vi "SW_BoolArryToNumber2.vi"(8 "error in (no error)":errorcluster caption="错误输入（无错误）", 10 "L32 INUPT":string="1.0.0.0", 11 "H32 INUPT":string="2.0.0.0") -> (0 "error out":errorcluster caption="错误输出", 1 "64 SW OUT":bool[](array[boolean]), 2 "L_32":bool[](array[boolean]), 3 "H_32":bool[](array[boolean]))   [LabVIEW 2018]
panel:
  out "数组 2":string[](array[string])
  out "数组":string[](array[string])
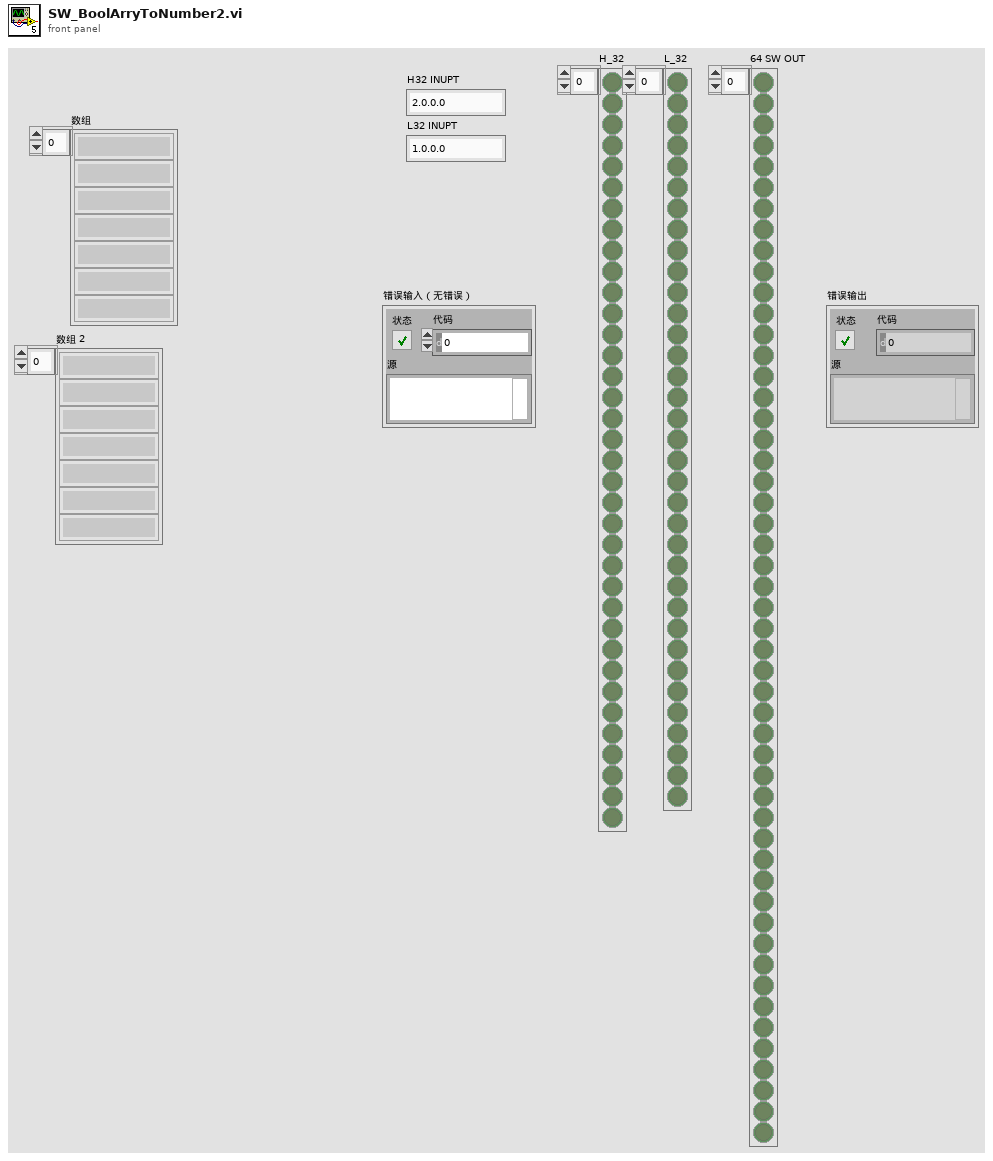
[diagram p1: front panel]
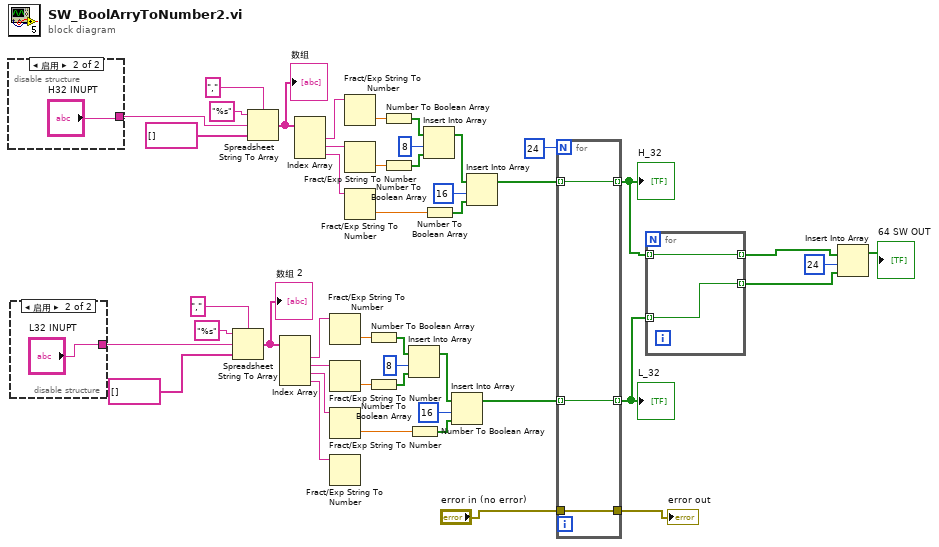
[diagram p0: block diagram]
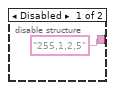
[diagram p2: hidden frame]
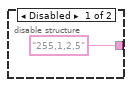
[diagram p3: hidden frame]
diagram:
  n1 = disable-structure shown="启用" {
    disable-tunnel: ["255,1,2,5" "H32 INUPT"] -> w44
    frame Disabled {
    }
    frame Enabled {
    }
  }
  n2 = disable-structure shown="启用" {
    disable-tunnel: ["255,1,2,5" "L32 INUPT"] -> w12
    frame Disabled {
    }
    frame Enabled {
    }
  }
  n3 = Spreadsheet String To Array(delimiter (Tab)="," ("分隔符(Tab)"), format string="%s" ("格式字符串"), spreadsheet string=w12, array type (2D Dbl)=string[] []) -> (array=w15:string[])
  "数组 2" <- w15
  n4 = Spreadsheet String To Array(delimiter (Tab)="," ("分隔符(Tab)"), format string="%s" ("格式字符串"), spreadsheet string=w44, array type (2D Dbl)=string[] []) -> (array=w42:string[])
  "数组" <- w42
  n5 = Index Array(array=w15) -> (element #1=w16:string, element #2=w18:string, element #3=w19:string, element #4=w20:string)  [unwired: 4 in]
  n6 = Index Array(array=w42) -> (element #1=w41:string, element #2=w39:string, element #3=w38:string)  [unwired: 3 in]
  n7 = Fract/Exp String To Number(string=w16) -> (number=w17:dbl)  [unwired: 3 in, 1 out]
  n8 = Fract/Exp String To Number(string=w18) -> (number=w21:dbl)  [unwired: 3 in, 1 out]
  n9 = Fract/Exp String To Number(string=w19) -> (number=w22:dbl)  [unwired: 3 in, 1 out]
  n10 = Fract/Exp String To Number(string=w20) -> ()  [unwired: 3 in, 2 out]
  n11 = Fract/Exp String To Number(string=w41) -> (number=w40:dbl)  [unwired: 3 in, 1 out]
  n12 = Fract/Exp String To Number(string=w39) -> (number=w37:dbl)  [unwired: 3 in, 1 out]
  n13 = Fract/Exp String To Number(string=w38) -> (number=w36:dbl)  [unwired: 3 in, 1 out]
  n14 = Number To Boolean Array(number=w17) -> (Boolean array=w23:bool[])
  n15 = Number To Boolean Array(number=w21) -> (Boolean array=w25:bool[])
  n16 = Number To Boolean Array(number=w40) -> (Boolean array=w35:bool[])
  n17 = Number To Boolean Array(number=w37) -> (Boolean array=w33:bool[])
  n18 = Insert Into Array(array=w23, index=8 ("索引"), new element=w25) -> (w27:bool[])
  n19 = Number To Boolean Array(number=w22) -> (Boolean array=w28:bool[])
  n20 = Insert Into Array(array=w35, index=8 ("索引"), new element=w33) -> (w31:bool[])
  n21 = Number To Boolean Array(number=w36) -> (Boolean array=w30:bool[])
  n22 = Insert Into Array(array=w27, index=16 ("索引"), new element=w28) -> (w1:bool[])
  n23 = Insert Into Array(array=w31, index=16 ("索引"), new element=w30) -> (w2:bool[])
  n24 = for {
    N: 24 -> [_]
    tunnel: w2 -> [w53] mode=indexing
    tunnel: [w53] -> w7 mode=indexing
    tunnel: w1 -> [w52] mode=indexing
    tunnel: [w52] -> w5 mode=indexing
    tunnel: [w51] -> w10
    tunnel: "error in (no error)" -> [w51]
  }
  "H_32" <- w7
  "L_32" <- w5
  "error out" <- w10
  n25 = for {
    tunnel: w7 -> [w55] mode=indexing
    tunnel: [w55] -> w6 mode=indexing
    tunnel: w5 -> [w54] mode=indexing
    tunnel: [w54] -> w4 mode=indexing
  }
  n26 = Insert Into Array(array=w6, index=24 ("索引"), new element=w4) -> (→"64 SW OUT":bool[])
